vi "Func-엑셀 데이터를 그래프로 출력.vi"() -> ()   [LabVIEW 2015] (continued)
89.43\n85\t85\t89.426\n85\t85\t89.426\n85\t85\t89.423\n85\t85\t89.423\n85\t85\t89.421\n85\t85\t89.425\n85\t85\t89.429\n85\t85\t89.43\n85\t85\t89.432\n85\t85\t89.433\n85\t85\t89.438\n85\t85\t89.436\n85\t85\t89.435\n85\t85\t89.434\n85\t85\t89.434\n85\t85\t89.433\n85\t85\t89.428\n85\t85\t89.432\n85\t85\t89.43\n85\t85\t89.428\n85\t85\t89.427\n85\t85\t89.432\n85\t85\t89.434\n85\t85\t89.433\n85\t85\t89.436\n85\t85\t89.439\n85\t85\t89.443\n85\t85\t89.437\n85\t85\t89.438\n85\t85\t89.437\n85\t85\t89.434\n85\t85\t89.434\n85\t85\t89.432\n85\t85\t89.434\n85\t85\t89.434\n85\t85\t89.431\n85\t85\t89.434\n85\t85\t89.437\n85\t85\t89.437\n85\t85\t89.438\n85\t85\t89.438\n85\t85\t89.439\n85\t85\t89.439\n85\t85\t89.436\n85\t85\t89.436\n85\t85\t89.436\n85\t85\t89.438\n85\t85\t89.439\n85\t85\t89.441\n85\t85\t89.441\n85\t85\t89.438\n85\t85\t89.439\n85\t85\t89.439\n85\t85\t89.441\n85\t85\t89.436\n85\t85\t89.432\n85\t85\t89.432\n85\t85\t89.434\n85\t85\t89.433\n85\t85\t89.43\n85\t85\t89.437\n85\t85\t89.439\n85\t85\t89.437\n85\t85\t89.437\n85\t85\t89.434\n85\t85\t89.435\n85\t85\t89.434\n85\t85\t89.436\n85\t85\t89.439\n85\t85\t89.437\n85\t85\t89.44\n85\t85\t89.438\n85\t85\t89.436\n85\t85\t89.435\n85\t85\t89.434\n85\t85\t89.432\n85\t85\t89.432\n85\t85\t89.435\n85\t85\t89.437\n85\t85\t89.44\n85\t85\t89.437\n85\t85\t89.44\n85\t85\t89.438\n85\t85\t89.439\n85\t85\t89.439\n85\t85\t89.443\n85\t85\t89.447\n85\t85\t89.446\n85\t85\t89.448\n85\t85\t89.446\n85\t85\t89.446\n85\t85\t89.441\n85\t85\t89.44\n85\t85\t89.442\n85\t85\t89.443\n85\t85\t89.445\n85\t85\t89.444\n85\t85\t89.448\n85\t85\t89.449\n85\t85\t89.448\n85\t85\t89.45\n85\t85\t89.445\n85\t85\t89.449\n85\t85\t89.448\n85\t85\t89.445\n85\t85\t89.446\n85\t85\t89.447\n85\t85\t89.447\n85\t85\t89.446\n85\t85\t89.445\n85\t85\t89.446\n85\t85\t89.448\n85\t85\t89.454\n85\t85\t89.454\n85\t85\t89.456\n85\t85\t89.454\n85\t85\t89.46\n85\t85\t89.459\n85\t85\t89.453\n85\t85\t89.455\n85\t85\t89.454\n85\t85\t89.451\n85\t85\t89.448\n85\t85\t89.447\n85\t85\t89.447\n85\t85\t89.446\n85\t85\t89.445\n85\t85\t89.452\n85\t85\t89.447\n85\t85\t89.449\n85\t85\t89.447\n85\t85\t89.445\n85\t85\t89.449\n85\t85\t89.447\n85\t85\t89.45\n85\t85\t89.454\n85\t85\t89.455\n85\t85\t89.454\n85\t85\t89.454\n85\t85\t89.454\n85\t85\t89.451\n85\t85\t89.45\n85\t85\t89.45\n85\t85\t89.452\n85\t85\t89.453\n85\t85\t89.454\n85\t85\t89.459\n85\t85\t89.459\n85\t85\t89.459\n85\t85\t89.46\n85\t85\t89.457\n85\t85\t89.459\n85\t85\t89.457\n85\t85\t89.457\n85\t85\t89.457\n85\t85\t89.457\n85\t85\t89.457\n85\t85\t89.454\n85\t85\t89.455\n85\t85\t89.453\n85\t85\t89.45\n85\t85\t89.45\n85\t85\t89.451\n85\t85\t89.453\n85\t85\t89.454\n85\t85\t89.454\n85\t85\t89.459\n85\t85\t89.462\n85\t85\t89.462\n85\t85\t89.465\n85\t85\t89.464\n85\t85\t89.465\n85\t85\t89.464\n85\t85\t89.46\n85\t85\t89.462\n85\t85\t89.461\n85\t85\t89.46\n85\t85\t89.457\n85\t85\t89.459\n85\t85\t89.46\n85\t85\t89.461\n85\t85\t89.459\n85\t85\t89.457\n85\t85\t89.462\n85\t85\t89.459\n85\t85\t89.459\n85\t85\t89.458\n85\t85\t89.462\n85\t85\t89.464\n85\t85\t89.463\n85\t85\t89.464\n85\t85\t89.462\n85\t85\t89.463\n85\t85\t89.459\n85\t85\t89.462\n85\t85\t89.466\n85\t85\t89.466\n85\t85\t89.466\n85\t85\t89.469\n85\t85\t89.472\n85\t85\t89.469\n85\t85\t89.466\n85\t85\t89.467\n85\t85\t89.467\n85\t85\t89.463\n85\t85\t89.462\n85\t85\t89.466\n85\t85\t89.463\n85\t85\t89.463\n85\t85\t89.466\n85\t85\t89.47\n85\t85\t89.47\n85\t85\t89.468\n85\t85\t89.474\n85\t85\t89.473\n85\t85\t89.474\n85\t85\t89.474\n85\t85\t89.477\n85\t85\t89.474\n85\t85\t89.468\n85\t85\t89.47\n85\t85\t89.469\n85\t85\t89.467\n85\t85\t89.466\n85\t85\t89.469\n85\t85\t89.476\n85\t85\t89.476\n85\t85\t89.477\n85\t85\t89.479\n85\t85\t89.48\n85\t85\t89.481\n85\t85\t89.474\n85\t85\t89.477\n85\t85\t89.477\n85\t85\t89.479\n85\t85\t89.479\n85\t85\t89.475\n85\t85\t89.481\n85\t85\t89.48\n85\t85\t89.484\n85\t85\t89.483\n85\t85\t89.48\n85\t85\t89.478\n85\t85\t89.484\n85\t85\t89.485\n85\t85\t89.479\n85\t85\t89.48\n85\t85\t89.483\n85\t85\t89.486\n85\t85\t89.481\n85\t85\t89.481\n85\t85\t89.483\n85\t85\t89.486\n85\t85\t89.487\n85\t85\t89.486\n85\t85\t89.488\n85\t85\t89.486\n85\t85\t89.485\n85\t85\t89.486\n85\t85\t89.49\n85\t85\t89.489\n85\t85\t89.491\n85\t85\t89.491\n85\t85\t89.493\n85\t85\t89.492\n85\t85\t89.486\n85\t85\t89.489\n85\t85\t89.485\n85\t85\t89.486\n85\t85\t89.485\n85\t85\t89.487\n85\t85\t89.486\n85\t85\t89.484\n85\t85\t89.483\n85\t85\t89.484\n85\t85\t89.484\n85\t85\t89.484\n85\t85\t89.487\n85\t85\t89.486\n85\t85\t89.49\n85\t85\t89.492\n85\t85\t89.496\n85\t85\t89.497\n85\t85\t89.494\n85\t85\t89.494\n85\t85\t89.493\n85\t85\t89.487\n85\t85\t89.48\n85\t85\t89.479\n85\t85\t89.477\n85\t85\t89.477\n85\t85\t89.48\n85\t85\t89.484\n85\t85\t89.484\n85\t85\t89.485\n85\t85\t89.486\n85\t85\t89.487\n85\t85\t89.487\n85\t85\t89.487\n85\t85\t89.489\n85\t85\t89.493\n85\t85\t89.494\n85\t85\t89.494\n85\t85\t89.495\n85\t85\t89.492\n85\t85\t89.492\n85\t85\t89.489\n85\t85\t89.493\n85\t85\t89.498\n85\t85\t89.503\n85\t85\t89.507\n85\t85\t89.508\n85\t85\t89.509\n85\t85\t89.507\n85\t85\t89.502\n85\t85\t89.498\n85\t85\t89.495\n85\t85\t89.496\n85\t85\t89.499\n85\t85\t89.5\n85\t85\t89.504\n85\t85\t89.502\n85\t85\t89.505\n85\t85\t89.507\n85\t85\t89.505\n85\t85\t89.508\n85\t85\t89.504\n85\t85\t89.507\n85\t85\t89.503\n85\t85\t89.505\n85\t85\t89.507\n85\t85\t89.504\n85\t85\t89.508\n85\t85\t89.504\n85\t85\t89.508\n85\t85\t89.504\n85\t85\t89.504\n85\t85\t89.503\n85\t85\t89.505\n85\t85\t89.51\n85\t85\t89.511\n85\t85\t89.514\n85\t85\t89.511\n85\t85\t89.516\n85\t85\t89.511\n85\t85\t89.51\n85\t85\t89.51\n85\t85\t89.509\n85\t85\t89.514\n85\t85\t89.511\n85\t85\t89.512\n85\t85\t89.509\n85\t85\t89.511\n85\t85\t89.513\n85\t85\t89.51\n85\t85\t89.509\n85\t85\t89.508\n85\t85\t89.509\n85\t85\t89.509\n85\t85\t89.507\n85\t85\t89.506\n85\t85\t89.507\n85\t85\t89.513\n85\t85\t89.517\n85\t85\t89.517\n85\t85\t89.517\n85\t85\t89.52\n85\t85\t89.521\n85\t85\t89.516\n85\t85\t89.517\n85\t85\t89.518\n85\t85\t89.518\n85\t85\t89.518\n85\t85\t89.515\n85\t85\t89.518\n85\t85\t89.518\n85\t85\t89.519\n85\t85\t89.519\n85\t85\t89.517\n85\t85\t89.523\n85\t85\t89.521\n85\t85\t89.52\n85\t85\t89.519\n85\t85\t89.523\n85\t85\t89.525\n85\t85\t89.522\n85\t85\t89.523\n85\t85\t89.523\n85\t85\t89.522\n85\t85\t89.518\n85\t85\t89.515\n85\t85\t89.517\n85\t85\t89.516\n85\t85\t89.516\n85\t85\t89.512\n85\t85\t89.517\n85\t85\t89.52\n85\t85\t89.517\n85\t85\t89.521\n85\t85\t89.524\n85\t85\t89.524\n85\t85\t89.523\n85\t85\t89.525\n85\t85\t89.525\n85\t85\t89.524\n85\t85\t89.521\n85\t85\t89.524\n85\t85\t89.525\n85\t85\t89.521\n85\t85\t89.52\n85\t85\t89.519\n85\t85\t89.522\n85\t85\t89.523\n85\t85\t89.52\n85\t85\t89.523\n85\t85\t89.52\n85\t85\t89.52\n85\t85\t89.518\n85\t85\t89.52\n85\t85\t89.52\n85\t85\t89.52\n85\t85\t89.526\n85\t85\t89.527\n85\t85\t89.53\n85\t85\t89.53\n85\t85\t89.535\n85\t85\t89.535\n85\t85\t89.534\n85\t85\t89.535\n85\t85\t89.531\n85\t85\t89.528\n85\t85\t89.522\n85\t85\t89.525\n85\t85\t89.524\n85\t85\t89.525\n85\t85\t89.523\n85\t85\t89.526\n85\t85\t89.531\n85\t85\t89.527\n85\t85\t89.53\n85\t85\t89.526\n85\t85\t89.527\n85\t85\t89.528\n85\t85\t89.528\n85\t85\t89.535\n85\t85\t89.53\n85\t85\t89.536\n85\t85\t89.539\n85\t85\t89.541\n85\t85\t89.542\n85\t85\t89.538\n85\t85\t89.54\n85\t85\t89.537\n85\t85\t89.539\n85\t85\t89.541\n85\t85\t89.538\n85\t85\t89.541\n85\t85\t89.541\n85\t85\t89.544\n85\t85\t89.541\n85\t85\t89.534\n85\t85\t89.534\n85\t85\t89.532\n85\t85\t89.535\n85\t85\t89.531\n85\t85\t89.536\n85\t85\t89.541\n85\t85\t89.545\n85\t85\t89.545\n85\t85\t89.543\n85\t85\t89.546\n85\t85\t89.548\n85\t85\t89.547\n85\t85\t89.548\n85\t85\t89.546\n85\t85\t89.548\n85\t85\t89.55\n85\t85\t89.548\n85\t85\t89.549\n85\t85\t89.549\n85\t85\t89.548\n85\t85\t89.545\n85\t85\t89.545\n85\t85\t89.545\n85\t85\t89.543\n85\t85\t89.545\n85\t85\t89.546\n85\t85\t89.547\n85\t85\t89.547\n85\t85\t89.546\n85\t85\t89.551\n85\t85\t89.547\n85\t85\t89.55\n85\t85\t89.55\n85\t85\t89.551\n85\t85\t89.55\n85\t85\t89.545\n85\t85\t89.55\n85\t85\t89.555\n85\t85\t89.556\n85\t85\t89.554\n85\t85\t89.553\n85\t85\t89.553\n85\t85\t89.552\n85\t85\t89.55\n85\t85\t89.548\n85\t85\t89.548\n85\t85\t89.552\n85\t85\t89.553\n85\t85\t89.553\n85\t85\t89.553\n85\t85\t89.557\n85\t85\t89.558\n85\t85\t89.555\n85\t85\t89.556\n85\t85\t89.554\n85\t85\t89.555\n85\t85\t89.552\n85\t85\t89.552\n85\t85\t89.553\n85\t85\t89.55\n85\t85\t89.554\n85\t85\t89.553\n85\t85\t89.553\n85\t85\t89.555\n85\t85\t89.555\n85\t85\t89.559\n85\t85\t89.557\n85\t85\t89.556\n85\t85\t89.562\n85\t85\t89.561\n85\t85\t89.566\n85\t85\t89.563\n85\t85\t89.56\n85\t85\t89.562\n85\t85\t89.558\n85\t85\t89.557\n85\t85\t89.556\n85\t85\t89.555\n85\t85\t89.56\n85\t85\t89.559\n85\t85\t89.563\n85\t85\t89.563\n85\t85\t89.56\n85\t85\t89.561\n85\t85\t89.558\n85\t85\t89.56\n85\t85\t89.558\n85\t85\t89.559\n85\t85\t89.558\n85\t85\t89.562\n85\t85\t89.564\n85\t85\t89.565\n85\t85\t89.566\n85\t85\t89.565\n85\t85\t89.566\n85\t85\t89.561\n85\t85\t89.562\n85\t85\t89.562\n85\t85\t89.561\n85\t85\t89.563\n85\t85\t89.563\n85\t85\t89.569\n85\t85\t89.571\n85\t85\t89.572\n85\t85\t89.577\n85\t85\t89.579\n85\t85\t89.579\n85\t85\t89.579\n85\t85\t89.577\n85\t85\t89.575\n85\t85\t89.574\n85\t85\t89.571\n85\t85\t89.572\n85\t85\t89.571\n85\t85\t89.571\n85\t85\t89.575\n85\t85\t89.577\n85\t85\t89.576\n85\t85\t89.577\n85\t85\t89.574\n85\t85\t89.573\n85\t85\t89.57\n85\t85\t89.567\n85\t85\t89.569\n85\t85\t89.571\n85\t85\t89.569\n85\t85\t89.567\n85\t85\t89.568\n85\t85\t89.574\n85\t85\t89.576\n85\t85\t89.577\n85\t85\t89.581\n85\t85\t89.582\n85\t85\t89.579\n85\t85\t89.576\n85\t85\t89.574\n85\t85\t89.573\n85\t85\t89.572\n85\t85\t89.575\n85\t85\t89.578\n85\t85\t89.58\n85\t85\t89.577\n85\t85\t89.579\n85\t85\t89.583\n85\t85\t89.586\n85\t85\t89.586\n85\t85\t89.584\n85\t85\t89.584\n85\t85\t89.585\n85\t85\t89.584\n85\t85\t89.579\n85\t85\t89.577\n85\t85\t89.581\n85\t85\t89.578\n85\t85\t89.576\n85\t85\t89.574\n85\t85\t89.576\n85\t85\t89.577\n85\t85\t89.575\n85\t85\t89.58\n85\t85\t89.577\n85\t85\t89.578\n85\t85\t89.582\n85\t85\t89.584\n85\t85\t89.585\n85\t85\t89.585\n85\t85\t89.59\n85\t85\t89.594\n85\t85\t89.59\n85\t85\t89.588\n85\t85\t89.587\n85\t85\t89.59\n85\t85\t89.587\n85\t85\t89.586\n85\t85\t89.587\n85\t85\t89.59\n85\t85\t89.59\n85\t85\t89.589\n85\t85\t89.589\n85\t85\t89.587\n85\t85\t89.586\n85\t85\t89.582\n85\t85\t89.583\n85\t85\t89.582\n85\t85\t89.58\n85\t85\t89.58\n85\t85\t89.588\n85\t85\t89.588\n85\t85\t89.583\n85\t85\t89.584\n85\t85\t89.587\n85\t85\t89.591\n85\t85\t89.588\n85\t85\t89.59\n85\t85\t89.597\n85\t85\t89.594\n85\t85\t89.593\n85\t85\t89.593\n85\t85\t89.589\n85\t85\t89.59\n85\t85\t89.592\n85\t85\t89.592\n85\t85\t89.597\n85\t85\t89.593\n85\t85\t89.592\n85\t85\t89.592\n85\t85\t89.592\n85\t85\t89.594\n85\t85\t89.595\n85\t85\t89.601\n85\t85\t89.604\n85\t85\t89.605\n85\t85\t89.605\n85\t85\t89.605\n85\t85\t89.605\n85\t85\t89.603\n85\t85\t89.604\n85\t85\t89.606\n85\t85\t89.601\n85\t85\t89.606\n85\t85\t89.605\n85\t85\t89.598\n85\t85\t89.596\n85\t85\t89.596\n85\t85\t89.601\n85\t85\t89.599\n85\t85\t89.597\n85\t85\t89.599\n85\t85\t89.602\n85\t85\t89.601\n85\t85\t89.6\n85\t85\t89.596\n85\t85\t89.602\n85\t85\t89.608\n85\t85\t89.603\n85\t85\t89.604\n85\t85\t89.608\n85\t85\t89.604\n85\t85\t89.604\n85\t85\t89.605\n85\t85\t89.606\n85\t85\t89.61\n85\t85\t89.611\n85\t85\t89.613\n85\t85\t89.61\n85\t85\t89.61\n85\t85\t89.61\n85\t85\t89.606\n85\t85\t89.6\n85\t85\t89.599\n85\t85\t89.599\n85\t85\t89.598\n85\t85\t89.596\n85\t85\t89.594\n85\t85\t89.596\n85\t85\t89.599\n85\t85\t89.598\n85\t85\t89.6\n85\t85\t89.6\n85\t85\t89.602\n85\t85\t89.606\n85\t85\t89.606\n85\t85\t89.609\n85\t85\t89.613\n85\t85\t89.62\n85\t85\t89.62\n85\t85\t89.616\n85\t85\t89.617\n85\t85\t89.619\n85\t85\t89.619\n85\t85\t89.617\n85\t85\t89.616\n85\t85\t89.62\n85\t85\t89.619\n85\t85\t89.62\n85\t85\t89.617\n85\t85\t89.617\n85\t85\t89.619\n85\t85\t89.619\n85\t85\t89.618\n85\t85\t89.616\n85\t85\t89.615\n85\t85\t89.618\n85\t85\t89.617\n85\t85\t89.62\n85\t85\t89.62\n85\t85\t89.621\n85\t85\t89.622\n85\t85\t89.618\n85\t85\t89.618\n85\t85\t89.62\n85\t85\t89.62\n85\t85\t89.62\n85\t85\t89.624\n85\t85\t89.626\n85\t85\t89.629\n85\t85\t89.621\n85\t85\t89.62\n85\t85\t89.619\n85\t85\t89.616\n85\t85\t89.616\n85\t85\t89.615\n85\t85\t89.623\n85\t85\t89.625\n85\t85\t89.625\n85\t85\t89.624\n85\t85\t89.625\n85\t85\t89.625\n85\t85\t89.621\n85\t85\t89.622\n85\t85\t89.622\n85\t85\t89.625\n85\t85\t89.625\n85\t85\t89.627\n85\t85\t89.627\n85\t85\t89.625\n85\t85\t89.627\n85\t85\t89.625\n85\t85\t89.623\n85\t85\t89.621\n85\t85\t89.621\n85\t85\t89.621\n85\t85\t89.623\n85\t85\t89.623\n85\t85\t89.622\n85\t85\t89.621\n85\t85\t89.623\n85\t85\t89.626\n85\t85\t89.625\n85\t85\t89.623\n85\t85\t89.629\n85\t85\t89.633\n85\t85\t89.63\n85\t85\t89.628\n85\t85\t89.629\n85\t85\t89.633\n85\t85\t89.631\n85\t85\t89.627\n85\t85\t89.627\n85\t85\t89.629\n85\t85\t89.63\n85\t85\t89.627\n85\t85\t89.627\n85\t85\t89.632\n85\t85\t89.639\n85\t85\t89.638\n85\t85\t89.64\n85\t85\t89.64\n85\t85\t89.642\n85\t85\t89.636\n85\t85\t89.634\n85\t85\t89.641\n85\t85\t89.637\n85\t85\t89.634\n85\t85\t89.636\n85\t85\t89.637\n85\t85\t89.634\n85\t85\t89.629\n85\t85\t89.625\n85\t85\t89.63\n85\t85\t89.627\n85\t85\t89.626\n85\t85\t89.627\n85\t85\t89.625\n85\t85\t89.632\n85\t85\t89.631\n85\t85\t89.635\n85\t85\t89.635\n85\t85\t89.639\n85\t85\t89.643\n85\t85\t89.641\n85\t85\t89.641\n85\t85\t89.641\n85\t85\t89.642\n85\t85\t89.64\n85\t85\t89.637\n85\t85\t89.633\n85\t85\t89.633\n85\t85\t89.632\n85\t85\t89.633\n85\t85\t89.632\n85\t85\t89.634\n85\t85\t89.635\n85\t85\t89.637\n85\t85\t89.641\n85\t85\t89.643\n85\t85\t89.644\n85\t85\t89.643\n85\t85\t89.644\n85\t85\t89.64\n85\t85\t89.634\n85\t85\t89.633\n85\t85\t89.632\n85\t85\t89.633\n85\t85\t89.633\n85\t85\t89.636\n85\t85\t89.64\n85\t85\t89.644\n85\t85\t89.643\n85\t85\t89.639\n85\t85\t89.639\n85\t85\t89.637\n85\t85\t89.637\n85\t85\t89.635\n85\t85\t89.641\n85\t85\t89.646\n85\t85\t89.651\n85\t85\t89.65\n85\t85\t89.651\n85\t85\t89.65\n85\t85\t89.641\n85\t85\t89.64\n85\t85\t89.636\n85\t85\t89.641\n85\t85\t89.641\n85\t85\t89.64\n85\t85\t89.645\n85\t85\t89.646\n85\t85\t89.653\n85\t85\t89.65\n85\t85\t89.648\n85\t85\t89.652\n85\t85\t89.652\n85\t85\t89.648\n85\t85\t89.646\n85\t85\t89.649\n85\t85\t89.65\n85\t85\t89.646\n85\t85\t89.645\n85\t85\t89.648\n85\t85\t89.647\n85\t85\t89.646\n85\t85\t89.646\n85\t85\t89.649\n85\t85\t89.65\n85\t85\t89.652\n85\t85\t89.655\n85\t85\t89.659\n85\t85\t89.658\n85\t85\t89.657\n85\t85\t89.652\n85\t85\t89.647\n85\t85\t89.647\n85\t85\t89.648\n85\t85\t89.652\n85\t85\t89.655\n85\t85\t89.659\n85\t85\t89.663\n85\t85\t89.662\n85\t85\t89.659\n85\t85\t89.656\n85\t85\t89.658\n85\t85\t89.657\n85\t85\t89.657\n85\t85\t89.656\n85\t85\t89.658\n85\t85\t89.659\n85\t85\t89.658\n85\t85\t89.659\n85\t85\t89.659\n85\t85\t89.656\n85\t85\t89.657\n85\t85\t89.652\n85\t85\t89.656\n85\t85\t89.654\n85\t85\t89.655\n85\t85\t89.659\n85\t85\t89.657\n85\t85\t89.66\n85\t85\t89.657\n85\t85\t89.659\n85\t85\t89.659\n85\t85\t89.659\n85\t85\t89.66\n85\t85\t89.661\n85\t85\t89.664\n85\t85\t89.666\n85\t85\t89.666\n85\t85\t89.669\n85\t85\t89.669\n85\t85\t89.666\n85\t85\t89.663\n85\t85\t89.661\n85\t85\t89.662\n85\t85\t89.658\n85\t85\t89.661\n85\t85\t89.662\n85\t85\t89.664\n85\t85\t89.665\n85\t85\t89.665\n85\t85\t89.663\n85\t85\t89.66\n85\t85\t89.655\n85\t85\t89.655\n85\t85\t89.655\n85\t85\t89.657\n85\t85\t89.659\n85\t85\t89.657\n85\t85\t89.661\n85\t85\t89.66\n85\t85\t89.66\n85\t85\t89.661\n85\t85\t89.663\n85\t85\t89.665\n85\t85\t89.666\n85\t85\t89.669\n85\t85\t89.669\n85\t85\t89.668\n85\t85\t89.668\n85\t85\t89.67\n85\t85\t89.668\n85\t85\t89.667\n85\t85\t89.672\n85\t85\t89.672\n85\t85\t89.672\n85\t85\t89.668\n85\t85\t89.67\n85\t85\t89.67\n85\t85\t89.663\n85\t85\t89.66\n85\t85\t89.661\n85\t85\t89.67\n85\t85\t89.668\n85\t85\t89.668\n85\t85\t89.673\n85\t85\t89.672\n85\t85\t89.674\n85\t85\t89.663\n85\t85\t89.664\n85\t85\t89.665\n85\t85\t89.663\n85\t85\t89.666\n85\t85\t89.664\n85\t85\t89.668\n85\t85\t89.668\n85\t85\t89.668\n85\t85\t89.669\n85\t85\t89.667\n85\t85\t89.669\n85\t85\t89.673\n85\t85\t89.67\n85\t85\t89.669\n85\t85\t89.667\n85\t85\t89.669\n85\t85\t89.668\n85\t85\t89.665\n85\t85\t89.671\n85\t85\t89.678\n85\t85\t89.682\n85\t85\t89.684\n85\t85\t89.684\n85\t85\t89.683\n85\t85\t89.68\n85\t85\t89.677\n85\t85\t89.677\n85\t85\t89.679\n85\t85\t89.68\n85\t85\t89.682\n85\t85\t89.683\n85\t85\t89.68\n85\t85\t89.679\n85\t85\t89.677\n85\t85\t89.675\n85\t85\t89.674\n85\t85\t89.673\n85\t85\t89.679\n85\t85\t89.682\n85\t85\t89.681\n85\t85\t89.681\n85\t85\t89.68\n85\t85\t89.679\n85\t85\t89.677\n85\t85\t89.677\n85\t85\t89.678\n85\t85\t89.676\n85\t85\t89.679\n85\t85\t89.68\n85\t85\t89.679\n85\t85\t89.677\n85\t85\t89.677\n85\t85\t89.677\n85\t85\t89.677\n85\t85\t89.673\n85\t85\t89.671\n85\t85\t89.67\n85\t85\t89.67\n85\t85\t89.673\n85\t85\t89.675\n85\t85\t89.675\n85\t85\t89.677\n85\t85\t89.677\n85\t85\t89.677\n85\t85\t89.678\n85\t85\t89.677\n85\t85\t89.679\n85\t85\t89.682\n85\t85\t89.685\n85\t85\t89.684\n85\t85\t89.682\n85\t85\t89.679\n85\t85\t89.682\n85\t85\t89.685\n85\t85\t89.683\n85\t85\t89.684\n85\t85\t89.687\n85\t85\t89.693\n85\t85\t89.694\n85\t85\t89.689\n85\t85\t89.688\n85\t85\t89.691\n85\t85\t89.69\n85\t85\t89.686\n85\t85\t89.681\n85\t85\t89.679\n85\t85\t89.683\n85\t85\t89.68\n85\t85\t89.681\n85\t85\t89.68\n85\t85\t89.68\n85\t85\t89.683\n85\t85\t89.682\n85\t85\t89.687\n85\t85\t89.686\n85\t85\t89.688\n85\t85\t89.696\n85\t85\t89.696\n85\t85\t89.695\n85\t85\t89.692\n85\t85\t89.693\n85\t85\t89.694\n85\t85\t89.69\n85\t85\t89.693\n85\t85\t89.691\n85\t85\t89.688\n85\t85\t89.686\n85\t85\t89.693\n85\t85\t89.693\n85\t85\t89.691\n85\t85\t89.689\n85\t85\t89.693\n85\t85\t89.693\n85\t85\t89.686\n85\t85\t89.688\n85\t85\t89.688\n85\t85\t89.689\n85\t85\t89.687\n85\t85\t89.692\n85\t85\t89.689\n85\t85\t89.689\n85\t85\t89.693\n85\t85\t89.695\n85\t85\t89.693\n85\t85\t89.692\n85\t85\t89.695\n85\t85\t89.694\n85\t85\t89.688\n85\t85\t89.687\n85\t85\t89.687\n85\t85\t89.69\n85\t85\t89.688\n85\t85\t89.69\n85\t85\t89.698\n85\t85\t89.701\n85\t85\t89.703\n85\t85\t89.704\n85\t85\t89.706\n85\t85\t89.704\n85\t85\t89.698\n85\t85\t89.695\n85\t85\t89.698\n85\t85\t89.696\n85\t85\t89.694\n85\t85\t89.691\n85\t85\t89.696\n85\t85\t89.693\n85\t85\t89.688\n85\t85\t89.69\n85\t85\t89.695\n85\t85\t89.7\n85\t85\t89.698\n85\t85\t89.697\n85\t85\t89.698\n85\t85\t89.694\n85\t85\t89.694\n85\t85\t89.687\n85\t85\t89.692\n85\t85\t89.697\n85\t85\t89.696\n85\t85\t89.698\n85\t85\t89.696\n85\t85\t89.702\n85\t85\t89.698\n85\t85\t89.696\n85\t85\t89.699\n85\t85\t89.7\n85\t85\t89.703\n85\t85\t89.7\n85\t85\t89.698\n85\t85\t89.7\n85\t85\t89.699\n85\t85\t89.696\n85\t85\t89.693\n85\t85\t89.694\n85\t85\t89.695\n85\t85\t89.697\n85\t85\t89.698\n85\t85\t89.699\n85\t85\t89.703\n85\t85\t89.704\n85\t85\t89.707\n85\t85\t89.702\n85\t85\t89.703\n85\t85\t89.704\n85\t85\t89.703\n85\t85\t89.704\n85\t85\t89.705\n85\t85\t89.706\n85\t85\t89.712\n85\t85\t89.713\n85\t85\t89.719\n85\t85\t89.714\n85\t85\t89.712\n85\t85\t89.712\n85\t85\t89.709\n85\t85\t89.708\n85\t85\t89.701\n85\t85\t89.706\n85\t85\t89.706\n85\t85\t89.708\n85\t85\t89.701\n85\t85\t89.702\n85\t85\t89.705\n85\t85\t89.704\n85\t85\t89.701\n85\t85\t89.701\n85\t85\t89.706\n85\t85\t89.707\n85\t85\t89.702\n85\t85\t89.705\n85\t85\t89.709\n85\t85\t89.713\n85\t85\t89.71\n85\t85\t89.709\n85\t85\t89.711\n85\t85\t89.709\n85\t85\t89.707\n85\t85\t89.703\n85\t85\t89.702\n85\t85\t89.706\n85\t85\t89.71\n85\t85\t89.714\n85\t85\t89.713\n85\t85\t89.718\n85\t85\t89.721\n85\t85\t89.718\n85\t85\t89.715\n85\t85\t89.715\n85\t85\t89.716\n85\t85\t89.71\n85\t85\t89.712\n85\t85\t89.712\n85\t85\t89.712\n85\t85\t89.709\n85\t85\t89.71\n85\t85\t89.707\n85\t85\t89.704\n85\t85\t89.707\n85\t85\t89.707\n85\t85\t89.707\n85\t85\t89.709\n85\t85\t89.713\n85\t85\t89.717\n85\t85\t89.716\n85\t85\t89.72\n85\t85\t89.718\n85\t85\t89.718\n85\t85\t89.719\n85\t85\t89.717\n85\t85\t89.716\n85\t85\t89.712\n85\t85\t89.714\n85\t85\t89.713\n85\t85\t89.711\n85\t85\t89.713\n85\t85\t89.713\n85\t85\t89.716\n85\t85\t89.713\n85\t85\t89.718\n85\t85\t89.718\n85\t85\t89.716\n85\t85\t89.717\n85\t85\t89.718\n85\t85\t89.718\n85\t85\t89.716\n85\t85\t89.718\n85\t85\t89.718\n85\t85\t89.716\n85\t85\t89.709
